vi "Symphony AverageDatOld.vi"(8 "error in (no error)":errorcluster caption="entrée d'erreur (pas d'erreur)", 10 "Image Mode":bool, 11 "RawDataIn":i32[][](array[numeric])) -> (0 "error out":errorcluster caption="sortie d'erreur", 3 "TableauOut":dbl[][](array[numeric]))   [LabVIEW 2019]
panel:
  in  "Noise Substract":bool
  in  "Column":i32
  in  "Row":i32
  in  "Page":i32
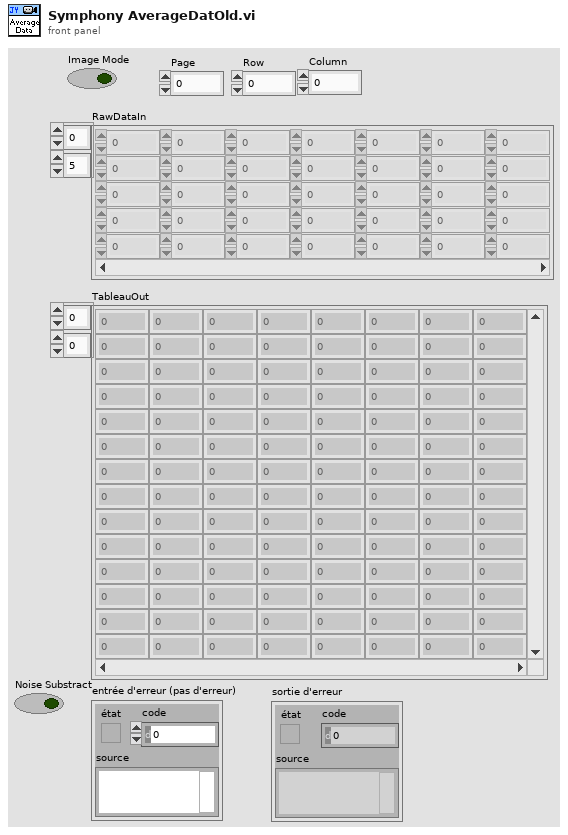
[diagram p1: front panel]
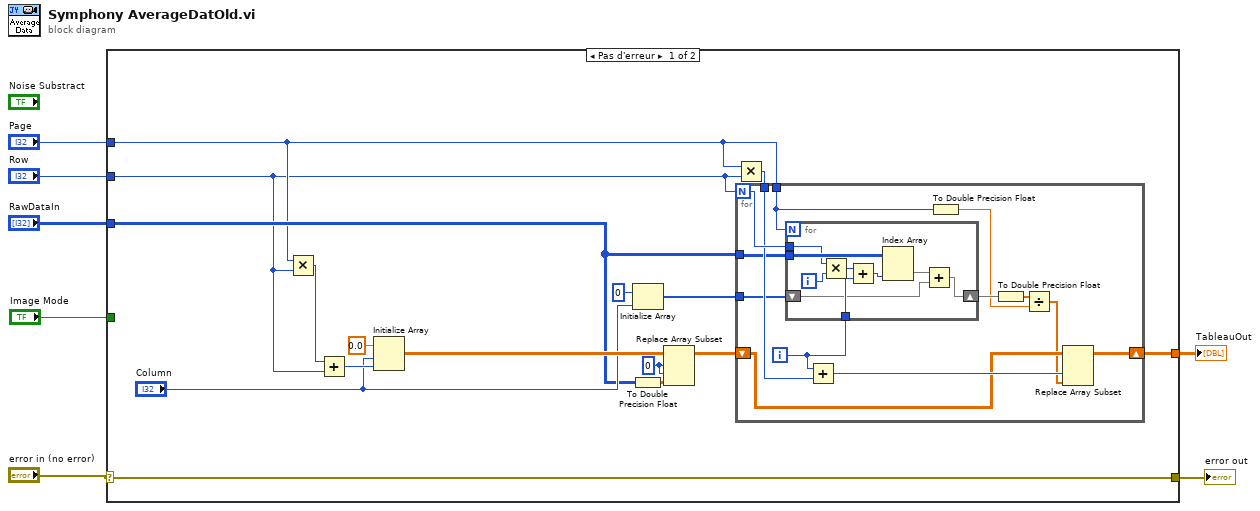
[diagram p0: block diagram]
diagram:
  n1 = case shown="Pas d'erreur" "error in (no error)" {
    selector: "error in (no error)" -> [w13 w46]
    tunnel: "Image Mode" -> [_ _]
    tunnel: "RawDataIn" -> [w11 _]
    tunnel: [w15 _] -> w5
    tunnel: [w13 w46] -> w3
    tunnel: "Page" -> [w9 _]
    tunnel: "Row" -> [w8 _]
    frame No Error {
      w16 = 0 ("indice (ligne)")
      n2 = Multiply(x=w9, y=w8) -> (x*y=w10:i32)
      n3 = Add(x=w10, y=w8) -> (x+y=w19:i32)
      n4 = Initialize Array(0.0 ("élément"), "Column", w19) -> (w18:dbl[][])
      n5 = Initialize Array(0 ("élément"), "Column") -> (w21:i32[])
      n6 = To Double Precision Float(number=w11) -> (double precision float=w14:dbl[][])
      n7 = Replace Array Subset(array=w18, new element=w14, index (row)=w16, index (col)=w16) -> (w17:dbl[][])
      n8 = Multiply(x=w9, y=w8) -> (x*y=w23:i32)
      n9 = for {
        N: w8 -> [w36]
        tunnel: w9 -> [w25]
        tunnel: w23 -> [w34]
        tunnel: w21 -> [w30]
        shift-right: [w28] -> w15
        shift-left: w17 -> [w29]
        tunnel: w11 -> [w33]
        i -> [w35]
        n10 = for {
          N: w25 -> [_]
          tunnel: w36 -> [w43]
          tunnel: w35 -> [w41]
          shift-right: [w38] -> w32
          shift-left: w30 -> [w37]
          tunnel: w33 -> [w44]
          i -> [w45]
          n11 = Multiply(x=w43, y=w45) -> (x*y=w42:i32)
          n12 = Add(x=w42, y=w41) -> (x+y=w40:i32)
          n13 = Index Array(array=w44, index (col)=w40) -> (element=w39:i32[])  [unwired: 1 in]
          n14 = Add(x=w39, y=w37) -> (x+y=w38:i32[])
        }
        n15 = Add(x=w35, y=w34) -> (x+y=w31:i32)
        n16 = To Double Precision Float(number=w25) -> (double precision float=w24:dbl)
        n17 = To Double Precision Float(number=w32) -> (double precision float=w26:dbl[])
        n18 = Divide(x=w26, y=w24) -> (x/y=w27:dbl[])
        n19 = Replace Array Subset(array=w29, new element=w27, index (col)=w31) -> (w28:dbl[][])  [unwired: 1 in]
      }
    }
    frame Error {
    }
  }
  "TableauOut" <- w5
  "error out" <- w3
